vi "Expand Alias Formula.vi"(11 "Alias Definition in":string) -> (3 "Expanded Alias Definition out":string)   [LabVIEW 2021, in "Formula.lvlib"]
uses:
  Formula.lvlib
  <userlib>/_OpenG.lib/array/array.llb/Reorder 1D Array2 (String)__ogtk.vi
  Strings/Strings.lvlib
  <userlib>/_OpenG.lib/array/array.llb/openg_array.lvlib
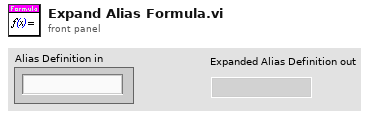
[diagram p1: front panel]
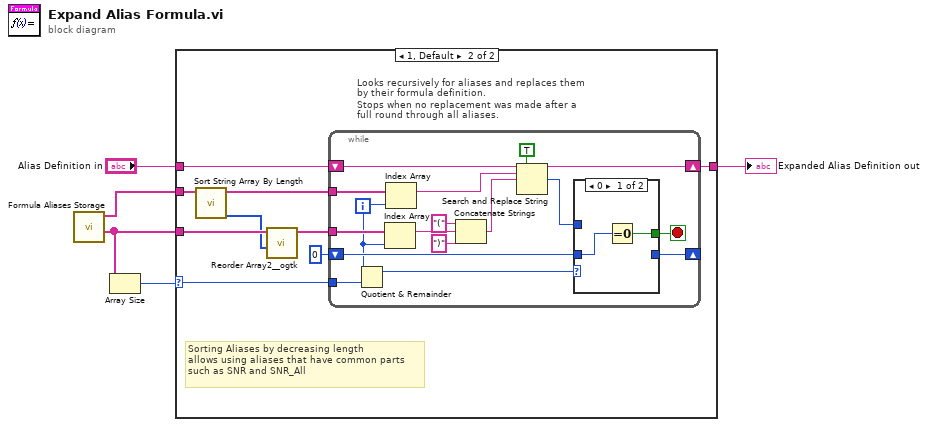
[diagram p0: block diagram]
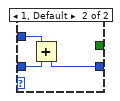
[diagram p3: hidden frame]
diagram:
  n1 = call "Formula Aliases Storage.vi"() -> ("Descriptions Array"=w3:string[], "Aliases Array"=w2:string[])  [unwired: 8 in, 2 out]
  n2 = Array Size(array=w3) -> (size(s)=w1:i32)
  n3 = case shown="1, Default" w1 {
    selector: w1 -> [_ w12]
    tunnel: "Alias Definition in" -> [w6 w15]
    tunnel: [w6 w14] -> w4
    tunnel: w3 -> [_ w9]
    tunnel: w2 -> [_ w11]
    frame 0 {
      # "No compound formula to analyze"
    }
    frame 1, Default {
      # "Sorting Aliases by decreasing length\nallows using aliases that have common parts\nsuch as SNR and SNR_All"
      n4 = call "Sort String Array By Length.vi"("String Array"=w11) -> ("Sorted Pointers"=w7:i32[], "Sorted String Array"=w10:string[])  [unwired: 9 in]
      n5 = call-poly <userlib>:"Reorder Array2__ogtk.vi"("indices"=w7, "array"=w9) -> ("reordered array"=w8:string[])  [unwired: 9 in]
      n6 = while "Looks recursively for aliases and replaces them by their formula definition.\nStops when no replacement was made after a full round through all aliases." {
        shift-right: [w31] -> w14
        shift-left: w15 -> [w32]
        tunnel: w10 -> [w30]
        tunnel: w8 -> [w29]
        shift-right: [w23] -> _
        shift-left: 0 -> [w25]
        tunnel: w12 -> [w21]
        i -> [w22]
        stop <- w19 stop-if-true
        n7 = Quotient & Remainder(x=w22, y=w21) -> (x-y*floor(x/y)=w20:i32)  [unwired: 1 out]
        n8 = Index Array(array=w29, index=w22) -> (element=w27:string)
        n9 = Index Array(array=w30, index=w22) -> (element=w28:string)
        n10 = Concatenate Strings("(" ("string"), w27, ")" ("string")) -> (w18:string)
        n11 = Search and Replace String(replace all?=TRUE ("replace all? (F)"), input string=w32, search string=w28, replace string=w18) -> (result string=w31:string, number of replacements=w26:i32)  [unwired: 4 in, 2 out]
        n12 = case shown="0" w20 {
          tunnel: w26 -> [_ w37]
          tunnel: w25 -> [w34 w36]
          tunnel: [_ w35] -> w23
          tunnel: [w33 _] -> w19
          frame 0 {
            n13 = Equal To 0?(x=w34) -> (x = 0?=w33:bool)
          }
          frame 1, Default {
            n14 = Add(x=w37, y=w36) -> (x+y=w35:i32)
          }
        }
      }
    }
  }
  "Expanded Alias Definition out" <- w4
